vi "TestingPolyFit.vi"() -> ()   [LabVIEW 2018]
uses:
  <vilib>/Analysis/NI_AALPro.lvlib
panel:
  out "Polynomial Coefficients":dbl[](array[numeric])
  out "Best Polynomial Fit":dbl[](array[numeric])
  out "XY Graph":cluster{dbl[], "Best Polynomial Fit":dbl[]}[](graph)
  in  "Random":dbl format="%#_13g"
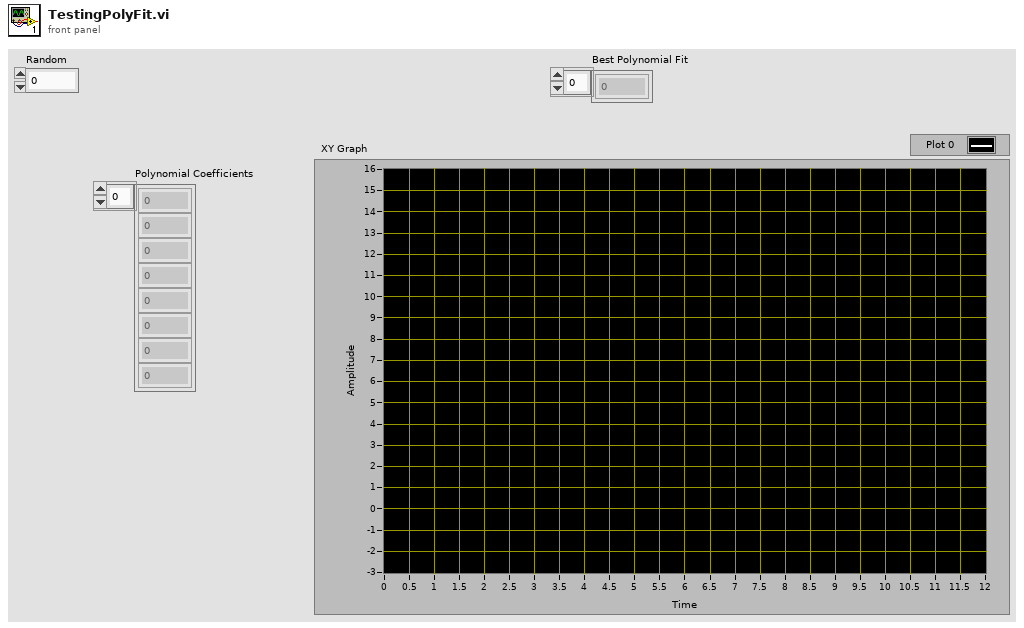
[diagram p1: front panel]
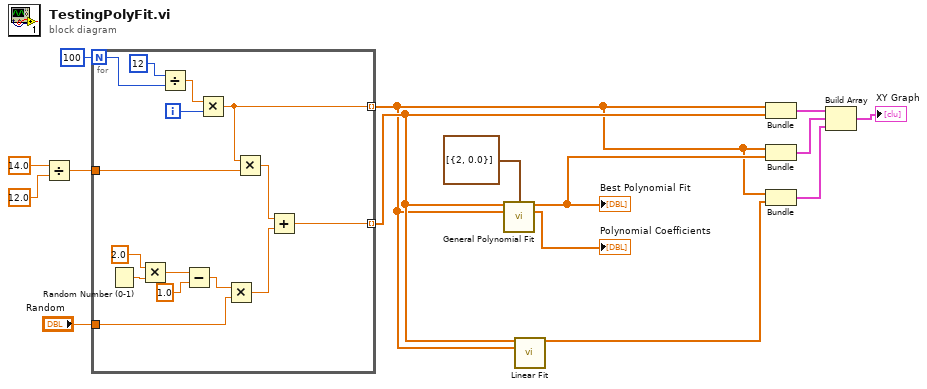
[diagram p0: block diagram]
diagram:
  n1 = Divide(x=14.0, y=12.0) -> (x/y=w12:dbl)
  n2 = for {
    N: 100 -> [w20]
    tunnel: w12 -> [w30]
    tunnel: "Random" -> [w24]
    tunnel: [w17] -> w4 mode=indexing
    tunnel: [w16] -> w3 mode=indexing
    i -> [w19]
    n3 = Random Number (0-1)() -> (number: 0 to 1=w29:dbl)
    n4 = Multiply(x=2.0, y=w29) -> (x*y=w27:dbl)
    n5 = Divide(x=12 ("y"), y=w20) -> (x/y=w18:dbl)
    n6 = Subtract(x=w27, y=1.0) -> (x-y=w25:dbl)
    n7 = Multiply(x=w18, y=w19) -> (x*y=w16:dbl)
    n8 = Multiply(x=w25, y=w24) -> (x*y=w23:dbl)
    n9 = Multiply(x=w16, y=w30) -> (x*y=w22:dbl)
    n10 = Add(x=w22, y=w23) -> (x+y=w17:dbl)
  }
  n11 = call <vilib>:"General Polynomial Fit.vi"("Y"=w4, "Coefficient Constraint"=cluster{"order":i32, "coefficient":dbl}[] [{"order"=2, "coefficient"=0.0}], "X"=w3) -> ("Best Polynomial Fit"=w9:dbl[], "Polynomial Coefficients"=→"Polynomial Coefficients":dbl[])  [unwired: 9 in, 2 out]
  "Best Polynomial Fit" <- w9
  n12 = call <vilib>:"Linear Fit.vi"("Y"=w4, "X"=w3) -> ("Best Linear Fit"=w2:dbl[])  [unwired: 9 in, 4 out]
  n13 = Bundle(w3, w4) -> (w8:cluster{dbl[], dbl[]})  [unwired: 1 in]
  n14 = Bundle(w3, "Best Polynomial Fit"=w9) -> (w7:cluster{dbl[], "Best Polynomial Fit":dbl[]})  [unwired: 1 in]
  n15 = Bundle(w3, "Best Linear Fit"=w2) -> (w1:cluster{dbl[], "Best Linear Fit":dbl[]})  [unwired: 1 in]
  n16 = Build Array(w8, w7, w1) -> (→"XY Graph":cluster{dbl[], "Best Linear Fit":dbl[]}[])
